vi "RM.getServerGUID.vi"(8 "error in (no error)":errorcluster, 11 "Item Ref in":T1 format="%.0x") -> (0 "error out":errorcluster, 1 "Found?":bool, 2 "ServerGUID":string, 3 "Item Ref out":T1 format="%.0x")   [LabVIEW 2016, in "FPGA Resource Manager.lvlib"]
uses:
  FPGA Resource Manager.lvlib
  <vilib>/NI Veristand/Custom Device API/Custom Device Item Ref.ctl
  RM.Globals.vi
  <vilib>/NI Veristand/Custom Device API/Get Item Property (String).vi
  <vilib>/NI Veristand/Custom Device API/Custom Device API.lvlib
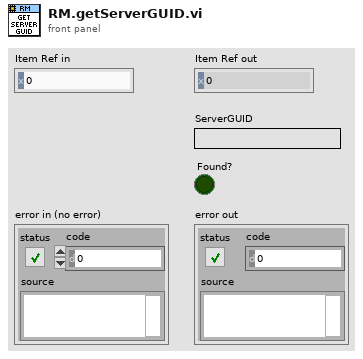
[diagram p1: front panel]
types:
  T1 = typedef "Custom Device API.lvlib/Custom Device Item Ref.ctl" = u64
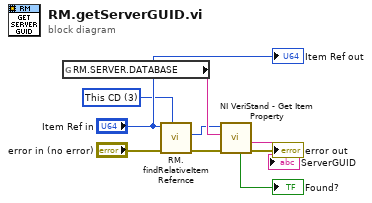
[diagram p0: block diagram]
diagram:
  w3 = u16 3 items=["Targets", "Controller", "Custom Devices", "This CD", "This CD/Group", "This CD/Group/SubGroup"] ("Relative Type")
  n1 = global read "RM.Globals.vi" "RM.SERVER.DATABASE"() -> (w7:string)
  n2 = call "RM.findRelativeItemRefernce.vi"("Relative Type"=w3, "error in (no error)"="error in (no error)", "Item Ref in"="Item Ref in") -> ("error out"=w6:errorcluster, "Relative Item Ref Out"=w5:T1)  [unwired: 4 in, 3 out]
  n3 = call-poly <vilib>:"NI VeriStand - Get Item Property.vi"("error in (no error)"=w6, "Property Name"=w7, "Item Ref in"=w5) -> ("error out"=→"error out":errorcluster, "Value"=→"ServerGUID":string, "Found?"=→"Found?":bool)  [unwired: 5 in, 1 out]
  "Item Ref out" <- "Item Ref in"
